vi "TEST_bench_FXP_Matrix-Vector_mult_loop_32bit.vi"(6 "NS + 1":u8=9, 8 "Az_col":fxp<+/-,32,5>[](array[numeric])=[0.0, 0.0, 0.0, 0.0, 0.0, 0.0, 0.0, 0.0, 0.0, 0.0, 0.0, 0.0, 0.0, 0.0, 0.0, 0.0, 0.0, 0.0, 0.0, 0.0, 0.0, 0.0, 0.0, 0.0, 0.0, 0.0, 0.0, 0.0, 0.0, 0.0, 0.0, 0.0, 0.0, 0.0, 0.0, 0.0, 0.0, 0.0, 0.0, 0.0, 0.0, 0.0, 0.0, 0.0, 0.0, 0.0, 0.0, 0.0, 0.0, 0.0], 11 "x_k":fxp<+/-,32,5>[](array[numeric])=[0.0, 0.0, 0.0, 0.0, 0.0, 0.0, 0.0, 0.0, 0.0, 0.0, 0.0, 0.0, 0.0, 0.0, 0.0, 0.0, 0.0, 0.0, 0.0, 0.0, 0.0, 0.0, 0.0, 0.0, 0.0, 0.0, 0.0, 0.0, 0.0, 0.0, 0.0, 0.0, 0.0, 0.0, 0.0, 0.0, 0.0, 0.0, 0.0, 0.0, 0.0, 0.0, 0.0, 0.0, 0.0, 0.0, 0.0, 0.0, 0.0, 0.0]) -> (3 "xk_1_0_mem":T1, 4 "xk_plus1":fxp<+/-,32,7>[](array[numeric]))   [LabVIEW 2017]
uses:
  fixed-point/typeDefs/x_vec_type.ctl
  fixed-point/typeDefs/x_vec_bram.ctl
  fixed-point/typeDefs/A_as_vec_bram.ctl
  <vilib>/rvi/DataTransferAndStorage/Container/Common/niFpgaContainerExecOnDevCompGetState.vi
  <vilib>/rvi/Emulation/niFpgaEmulationIsFPGAContextNoSignature.vi
  <vilib>/rvi/DataTransferAndStorage/Container/Common/niFpgaContainerGetUniqueNameForEmu.vi
  <vilib>/rvi/Emulation/niFpgaProcessEmulError.vi
  <vilib>/rvi/Emulation/niFpgaSctlEmulationGetInTimedLoop.vi
  <vilib>/rvi/errors/nirviReportUnexpectedCaseInternalError (U32).vi
  <vilib>/rvi/Memory/Memory_Emulation/niFpgaMemoryEmulationCacheClearOnFirstRun.vi
  <vilib>/rvi/Memory/Memory_Emulation/nirvimemoryEmulationManagerCache_MakeExclusive.vi
  <vilib>/rvi/Memory/Memory_Emulation/niFpgaMemoryEmulationValidateCache.vi
  <vilib>/rvi/Memory/Memory_Emulation/nirvimemoryEmulationManagerCache_InsertValue.vi
  <vilib>/Utility/error.llb/Clear Errors.vi
  <vilib>/rvi/Memory/Memory_Emulation/nirvimemoryEmulationManagerCache_ReleaseExclusive.vi
  <vilib>/rvi/Memory/Memory_Emulation/nirvimemoryEmulationManagerCache_GetValue.vi
  <vilib>/rvi/Memory/Memory_Emulation/nirvimemoryEmulationManagerCache_SetValue.vi
  <vilib>/rvi/Emulation/niFpgaSctlEmulationResourceMgr.vi
  <vilib>/rvi/DataTransferAndStorage/Container/XNode/niFpgaContainer.xnode
  <vilib>/rvi/Memory/Memory_Emulation/niFpgaMemoryEmulationRefIn.vi
panel:
  out "Array":fxp<+/-,32,6>[](array[numeric])
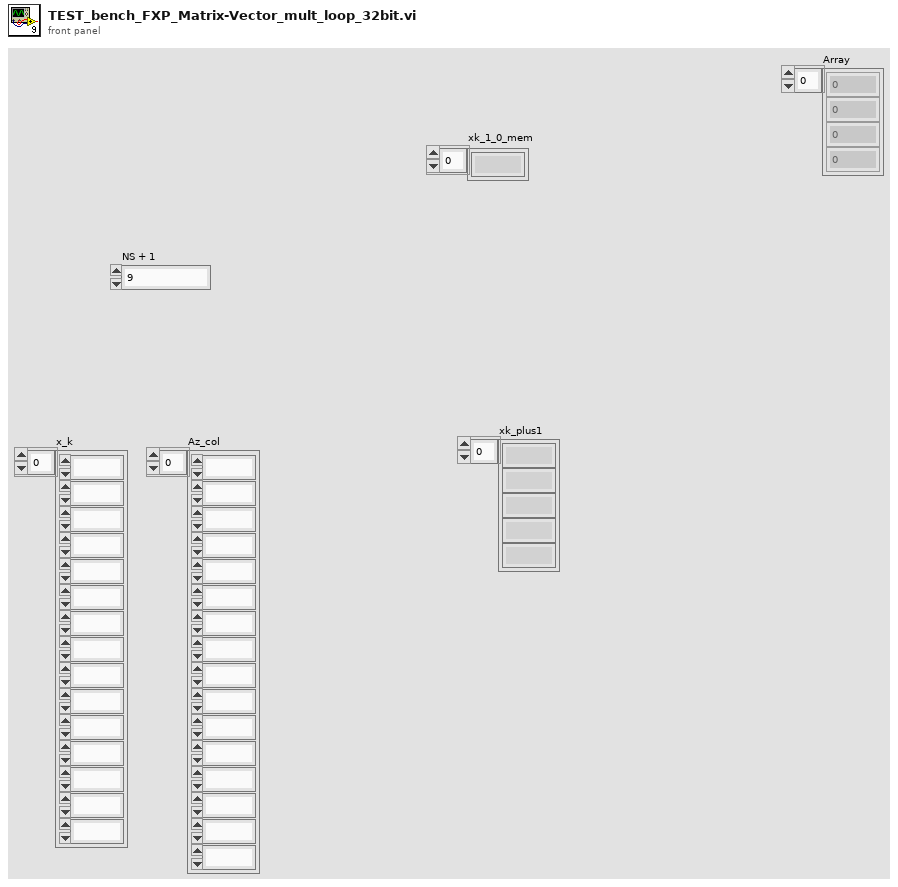
[diagram p1: front panel]
types:
  T1 = typedef "x_vec_type.ctl" = fxp<+/-,32,6>[]
  T2 = typedef "x_vec_bram.ctl" = refnum<k21>
  T3 = typedef "A_as_vec_bram.ctl" = refnum<k21>
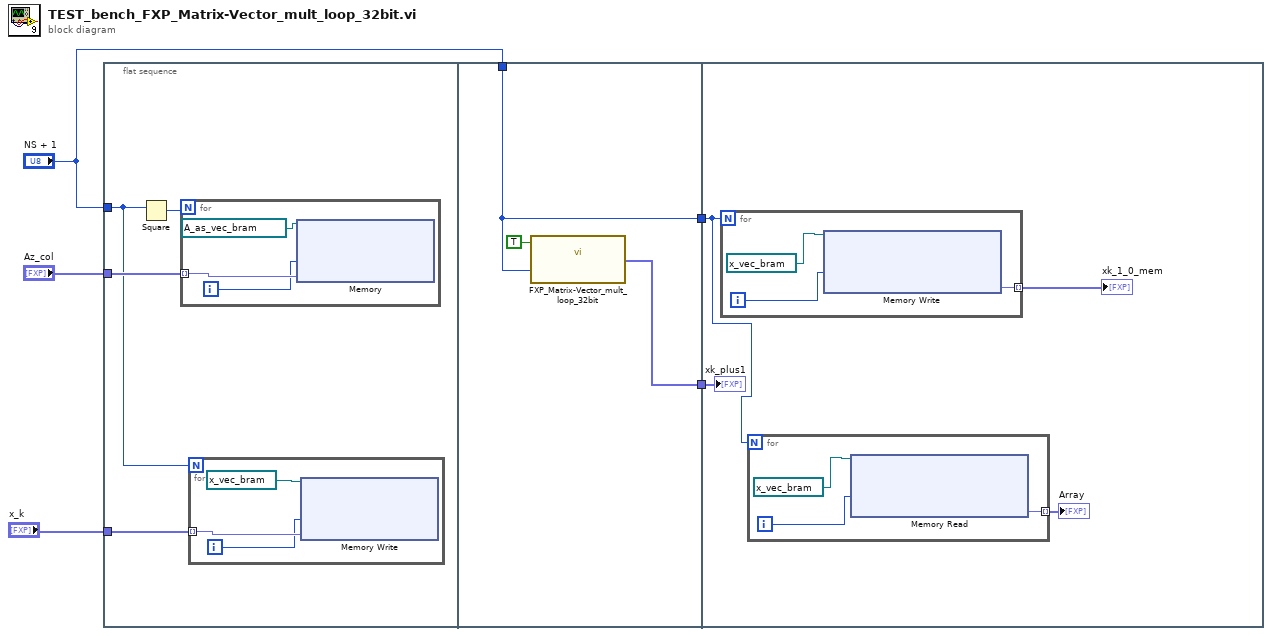
[diagram p0: block diagram]
diagram:
  n1 = flat-sequence {
    tunnel: "NS + 1" -> [w6]
    tunnel: "Az_col" -> [w9]
    tunnel: "x_k" -> [w8]
    tunnel: "NS + 1" -> [w18]
    tunnel: [w18] -> w2
    tunnel: [w16] -> w1
    tunnel: w2 -> [w20]
    tunnel: w1 -> [w22]
    frame #0 {
      n2 = Square(x=w6) -> (x^2=w7:u8)
      n3 = for {
        N: w7 -> [_]
        tunnel: w9 -> [w15] mode=indexing
        i -> [w14]
        n4 = xnode "Memory"("Address"=w14, "Data"=w15, "Memory In"=T3 "AasCol _FXP") -> ()  [unwired: 1 out]
      }
      n5 = for {
        N: w6 -> [_]
        tunnel: w8 -> [w12] mode=indexing
        i -> [w11]
        n6 = xnode "Memory Write"("Address"=w11, "Data"=w12, "Memory In"=T2 "xk_1_1" ("Memory")) -> ()  [unwired: 1 out]
      }
    }
    frame #1 {
      n7 = call "FXP_Matrix-Vector_mult_loop_32bit.vi"("Ns_2"=w18, "inputValid"=TRUE) -> ("Array"=w16:fxp<+/-,32,13>[])  [unwired: 9 in]
    }
    frame #2 {
      n8 = for {
        N: w20 -> [_]
        tunnel: [w27] -> w21 mode=indexing
        i -> [w28]
        n9 = xnode "Memory Write"("Address"=w28, "Memory In"=T2 "xk_1_0" ("Memory")) -> ("Data"=w27:fxp<+/-,32,6>)  [unwired: 1 out]
      }
      "xk_1_0_mem" <- w21
      n10 = for {
        N: w20 -> [_]
        tunnel: [w24] -> w19 mode=indexing
        i -> [w25]
        n11 = xnode "Memory Read"("Address"=w25, "Memory In"=T2 "xk_1_1" ("Memory")) -> ("Data"=w24:fxp<+/-,32,6>)  [unwired: 1 out]
      }
      "Array" <- w19
      "xk_plus1" <- w22
    }
  }
